vi "KPRO_2016_DPT.vi"() -> ()   [LabVIEW 2016]
uses:
  Kpro Globals.vi
  ad interface/Global_SIM_switch.vi
  <vilib>/Utility/file.llb/Write To Spreadsheet File (DBL).vi
panel:
  in  "Case Constant\n(See Context Help)":bool
  in  "Record DTW":bool
  out "Depth to Water":dbl=-30.877198474121087 format="%.2f"
  in  "In-Line Pressure Offset":dbl format="%.2f"
  in  "Zero In-Line Pressure\n(F = leave as is)":bool=TRUE
  in  "In-Line Pressure Slope":dbl=42.0 format="%.2f"
  out "In-Line Pressure":dbl=69.7228 format="%.2f"
  out "Drive Rate":dbl=16.666666666666664 format="%.2f"
  out "Real Time - Depth vs. Drive":cluster{dbl[], dbl[]}(graph)={[0.02036245163917736, 0.125, 0.16666666666666674, 0.16666666666666663, 0.16666666666666663, 0.16666666666666663], [-100.1, -100.2, -100.3, -100.4, -100.5, -100.6]}
  out "Current Depth (m)":sgl=-30.661383 format="%.2f"
  out "Zeroed \nPressure (m)":dbl=22.78027421497274 format="%.2f"
  out "Ik":dbl=0.003788962123473114 format="%.2f"
  in  "KPRO_test_report_header":string="Time(msecs)\tUncorrected_Depth\tCorrected_Depth\tDrive_Rate\tFlow\tFeet_of_Stainless\tPressure\tIK\tCorrected_Pressure\tAtm_Pressure\tDepth_to_water\tHeight_of_box\tRes_Pressure\tSecs_since_1_JAN_1904\tDepth_jumps_more_than_1_foot\r\n"
  in  "SLUG_test_report_header":string="Time(msecs)\tPressure\tFlow\n"
  in  "YSI_test_report_header":string="Depth\tPressure\tTemperature\tSpecific Conductivity\tDissolved O2\tPH\tOrp\tION\n"
  out "IK_for_GMS_report_header":string="Name\tHOLE_001\rXYZ\t20\t10\t30\rNumcols\t2\rNumrows\t1\rDepth\tIk\r"
  in  "Numrowswrite":string="1"
  in  "E":string="30"
  in  "Northing":string="10"
  in  "Easting":string="20"
  in  "Hole Id":string="HOLE_001"
  in  "Hole_name_file":path=path "C:/e"
  in  "Output File KPRO Test":path=path "C:/e_KPRO.txt"
  in  "Output File Slug Test":path=path "C:/e_SLUG.txt"
  in  "Output File YSI Test":path=path "C:/e_YSI.txt"
  in  "Output File IK for GMS":path=path "C:/e_IKMGS.txt"
  in  "enable_IKMGS_file":bool
  in  "enable_YSI_file":bool
  in  "enable_slug_file":bool
  in  "enable_kpro_file":bool=TRUE
  out "Ik":dbl=0.003788962123473114 format="%.2f"
  out "Zeroed Pressure":dbl=74.74207969932556 format="%.2f"
  out "Current Depth":sgl=-100.6 format="%.2f"
  out "Flow":dbl=0.21081600494384767 format="%.2f"
  out "Real Time - Depth vs. lk":cluster{dbl[], dbl[]}(graph)={[0.003788962123473114, 0.0037174584307500765, 0.0037174584307500765, 0.0037174584307500765, 0.0037174584307500765, 0.003788962123473114], [-100.1, -100.2, -100.3, -100.4, -100.5, -100.6]}
  out "Profile ID":string="WP-01"
  out "KPRO Box Number":dbl=800.0
  out "Last_String_Pot_Slope":dbl=1.6619999408721924 format="%.2f"
  out "Last_Flow_Slope":dbl=39.040000915527344 format="%.2f"
  out "Last_Pressure_Slope":dbl=48.27000045776367 format="%.2f"
  out "Height of Sample Box":dbl format="%.2f"
  out "Hole_Name_Path":path=path "C:/e"
  out "Cumulative_data_from_file":sgl[][](array[numeric]) format="%.2f"
  in  "data_directory":string="C:\\KPRO_DATA\\SITE_NAME\\"
  out "Cumulative_data_ready":bool
  out "Real Time - Depth vs. lk":cluster{dbl[], dbl[]}(graph)={[0.003788962123473114, 0.0037174584307500765, 0.0037174584307500765, 0.0037174584307500765, 0.0037174584307500765, 0.003788962123473114], [-100.1, -100.2, -100.3, -100.4, -100.5, -100.6]}
  in  "Reservoir Pressure":dbl=-0.004827000045779073 format="%.2f"
  in  "Simulate AD6B":bool
  in  "Atmospheric Pressure":dbl=32.22022530555725 format="%.2f"
  out "Depth to Water Table":dbl=-0.0 format="%.2f"
  in  "Ion Offset":dbl format="%.2f"
  in  "Ion Slope":dbl=44.04 format="%.2f"
  out "Pressure Slope":dbl=48.27000045776367 format="%.2f"
  out "Flow Slope":dbl=39.040000915527344 format="%.2f"
  out "String Pot Slope":dbl=1.6619999408721924 format="%.2f"
  in  "KPRO Com Port":i32=6
  in  "YSI Time Out (secs)":i32=5000
  in  "YSI Com Port":i32=7
  out "numrows":dbl format="%.2f"
  out "Slug Test\nIndicator copy":bool
  in  "ISE":bool=TRUE
  in  "Start\nYSI Capture":bool
  in  "Capture Head \nPressure":bool
  in  "Depth mode":bool caption="Use \nIncrement"
  out "Real Time - Depth vs. Drive":cluster{dbl[], dbl[]}(graph)={[0.02036245163917736, 0.125, 0.16666666666666674, 0.16666666666666663, 0.16666666666666663, 0.16666666666666663], [-100.1, -100.2, -100.3, -100.4, -100.5, -100.6]}
  out "Cumulative - Depth vs. Drive":cluster{dbl[], dbl[]}(graph)
  in  "Feet of Stainless":i32=40
  out "Zero Pressure\nIndicator":bool
  out "Slug Test\nIndicator":bool
  out "KPRO Test\nIndicator":bool
  in  "Increment\nButton":bool
  in  "Start\nST":bool
  in  "Zero\nPressure":bool
  out "Zeroed \nPressure":dbl=74.74207969932556 format="%.2f"
  in  "Finish Tests":bool
  out "Current Depth":sgl=-100.6 format="%.2f"
  in  "Start\nKPRO":bool
  out "Total Volume":dbl format="%.2f"
  in  "Clear \nTotal\nVolume":bool
  in  "Start Depth":sgl format="%.2f"
  in  "Client ID - Not Used":string
  out "Flow":dbl=0.21081600494384767 format="%.2f"
  out "Cumulative - Depth vs. Ik":cluster{dbl[], dbl[]}(graph)
  # "Use new slope/offset"
  # "KPRO  DATALOGGER"
  # "STONE  ENVIRONMENTAL  2010"
  # "ON"
  # "ON"
  # "OFF"
  # "OFF"
  # "ON"
  # "ON"
  # "OFF"
  # "OFF"
  # "ON"
  # "OFF"
  # "String Pot"
  # "Revision History\n\nAdded metric depth and pressure - VLD - 12-20-07\nAdded Static Ik button and drive rate- VLD 1-28-10"
  # "Use Incr"
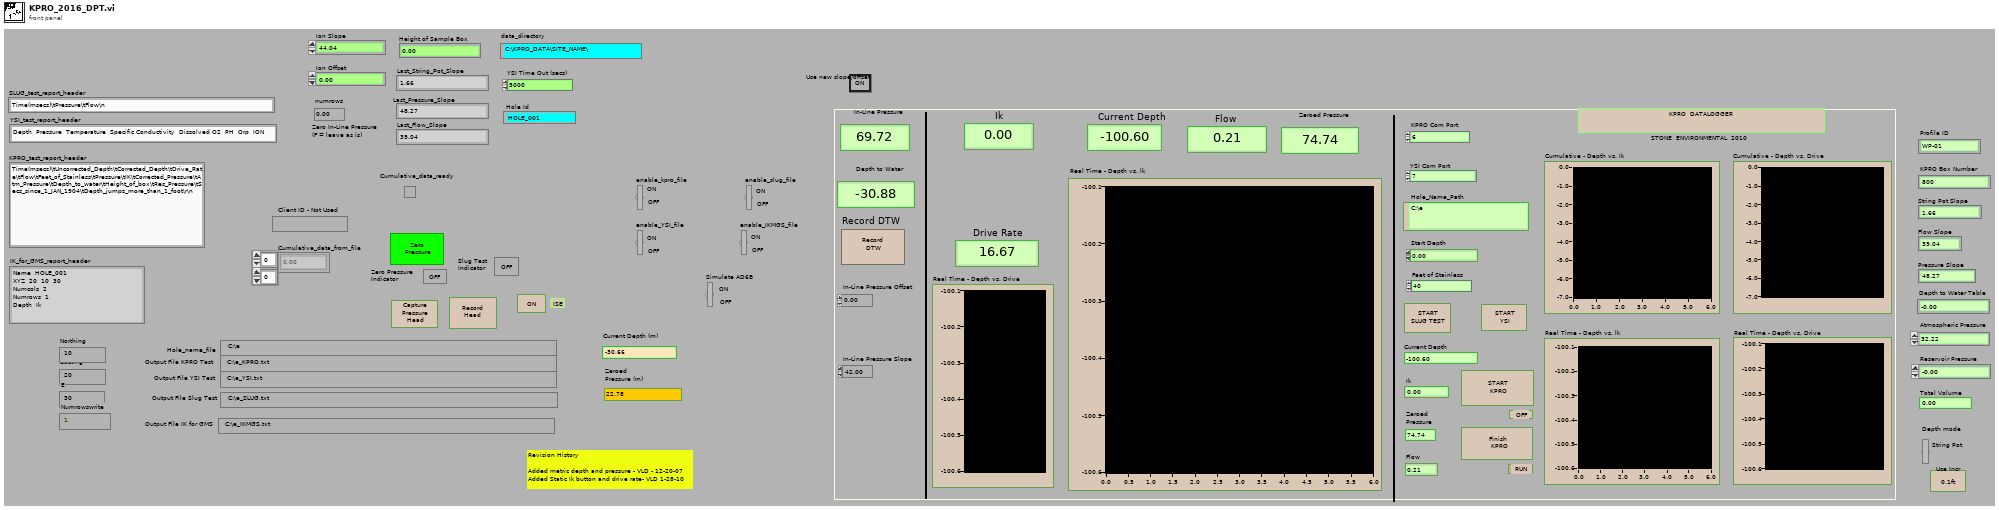
[diagram p1: front panel]
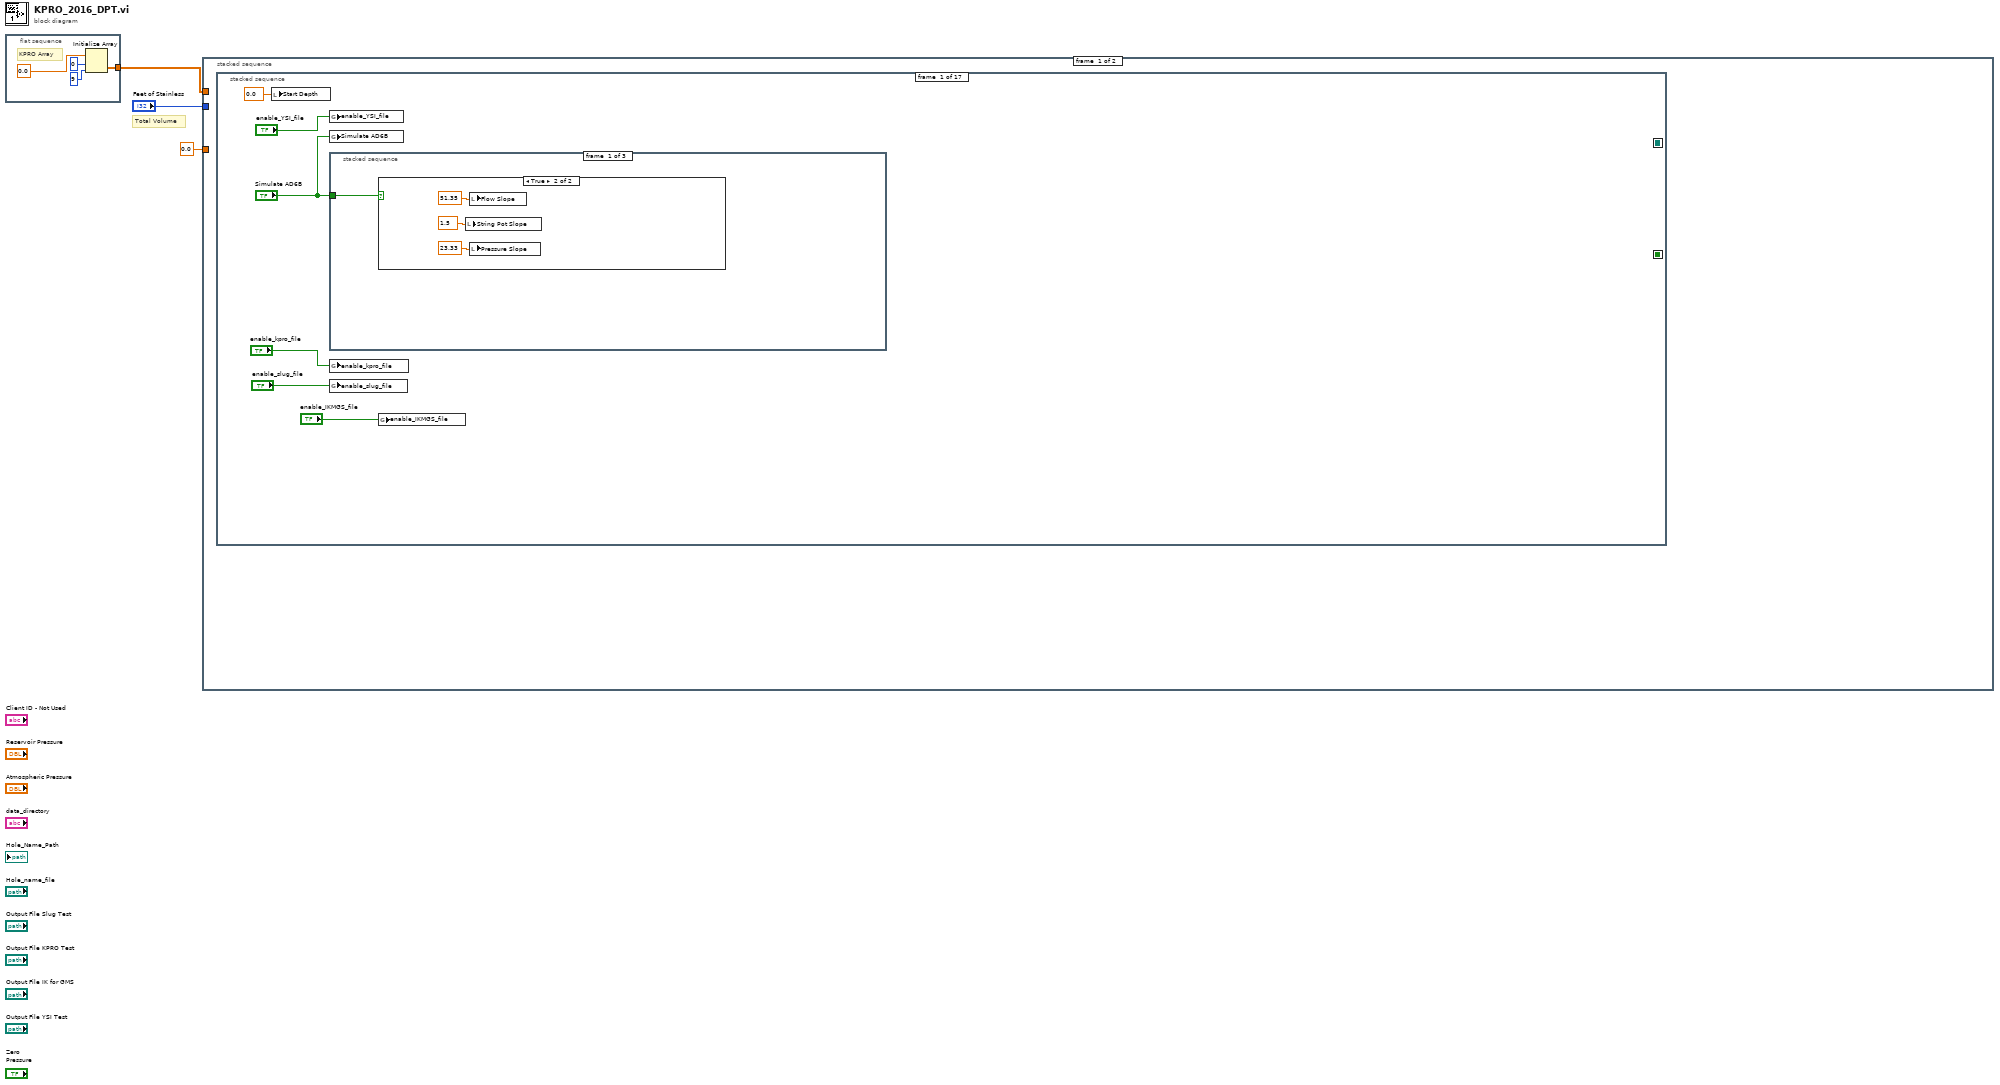
[diagram p0: block diagram]
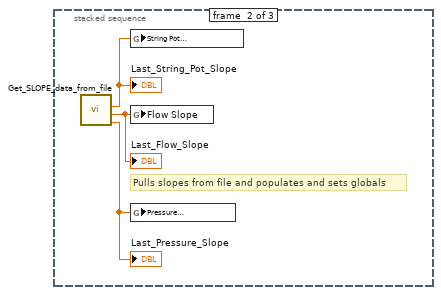
[diagram p3: hidden frame]
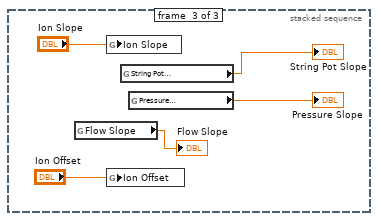
[diagram p4: hidden frame]
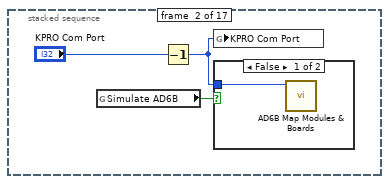
[diagram p5: hidden frame]
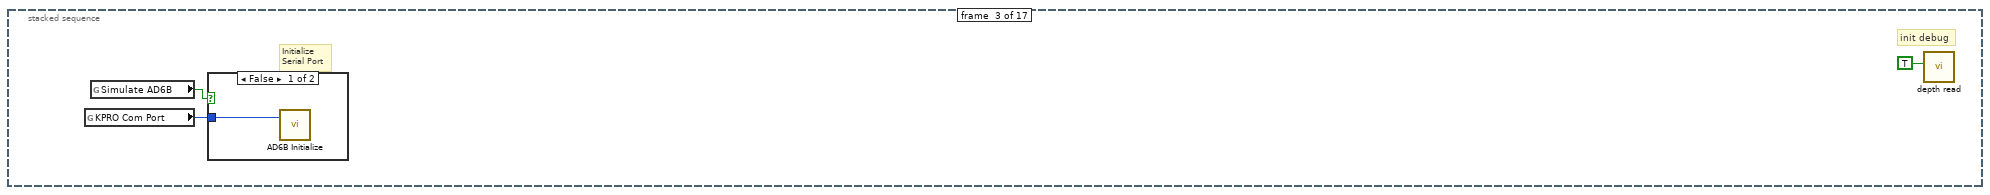
[diagram p7: hidden frame]
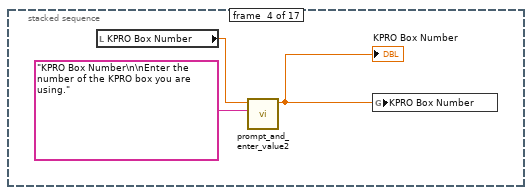
[diagram p9: hidden frame]
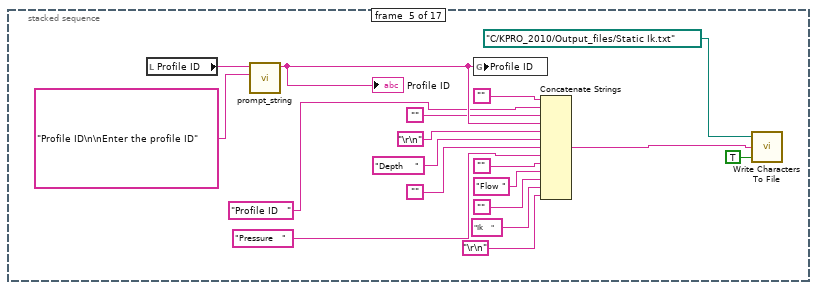
[diagram p10: hidden frame]
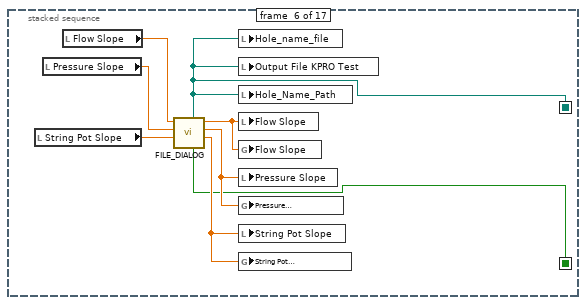
[diagram p11: hidden frame]
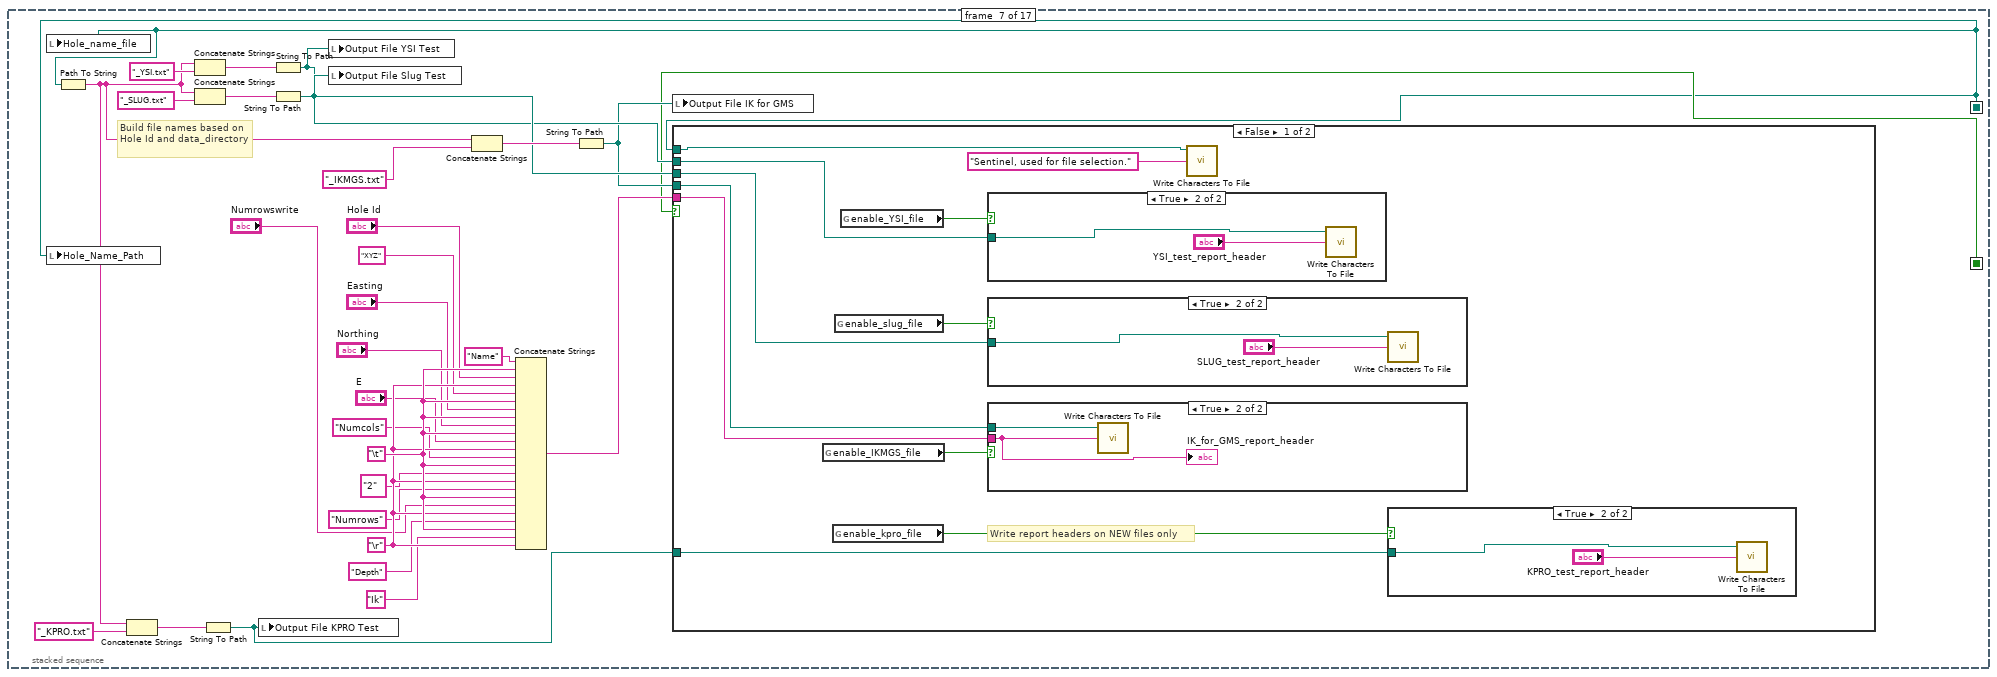
[diagram p12: hidden frame]
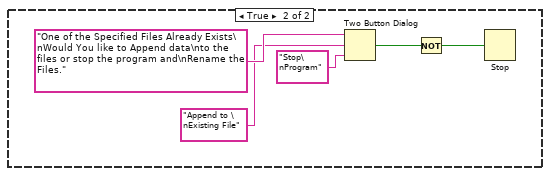
[diagram p17: hidden frame]
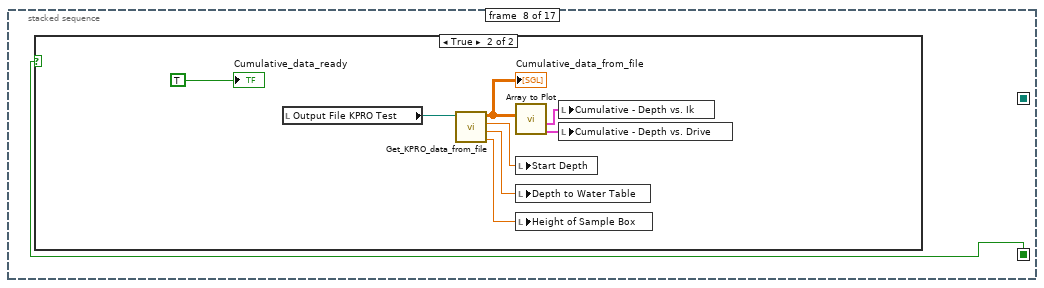
[diagram p18: hidden frame]
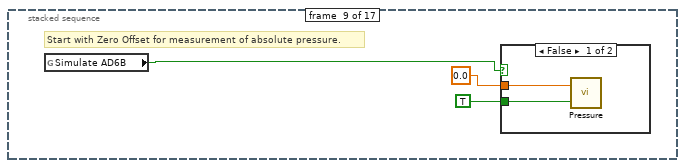
[diagram p20: hidden frame]
diagram:
  # "Total Volume"
  n1 = flat-sequence {
    tunnel: [w4] -> w1
    frame #0 {
      # "KPRO Array"
      n2 = Initialize Array(0.0, 0, 9) -> (w4:dbl[][])
    }
  }
  n3 = stacked-sequence {
    tunnel: "Feet of Stainless" -> [_ w195]
    tunnel: 0.0 -> [_ w194]
    tunnel: w1 -> [_ w193]
    frame #0 {
      n4 = stacked-sequence {
        seq-local: [_ _ _ _ _ w55 _ _ _ _ _ _ _ _ _ _ _] -> [_ _ _ _ _ _ w64 w117 _ _ _ _ _ _ _ _ _]
        seq-local: [_ _ _ _ _ w56 _ _ _ _ _ _ _ _ _ _ _] -> [_ _ _ _ _ _ w63 _ _ _ _ _ _ _ _ _ _]
        frame #0 {
          n5 = local write "Start Depth"(sgl 0.0 ("Start Depth")) -> ()
          n6 = global write "Global_SIM_switch.vi" "enable_YSI_file"("enable_YSI_file") -> ()
          n7 = global write "Global_SIM_switch.vi" "Simulate AD6B"("Simulate AD6B") -> ()
          n8 = stacked-sequence {
            tunnel: "Simulate AD6B" -> [w14 _ _]
            frame #0 {
              n9 = case shown="True" w14 {
                frame False {
                }
                frame True {
                  n10 = local write "String Pot Slope"(1.5 ("String Pot Slope")) -> ()
                  n11 = local write "Flow Slope"(51.35 ("Flow Slope")) -> ()
                  n12 = local write "Pressure Slope"(23.33 ("Pressure Slope")) -> ()
                }
              }
            }
            frame #1 {
              # "Pulls slopes from file and populates and sets globals"
              n13 = call "Get_SLOPE_data_from_file.vi"() -> ("Last_Pressure_Slope"=w20:dbl, "Last_Flow_Slope"=w19:dbl, "Last_String_Pot_Slope"=w18:dbl)  [unwired: 8 in, 1 out]
              "Last_Pressure_Slope" <- w20
              "Last_Flow_Slope" <- w19
              "Last_String_Pot_Slope" <- w18
              n14 = global write "Kpro Globals.vi" "String Pot \nSlope"(w18) -> ()
              n15 = global write "Kpro Globals.vi" "Flow Slope"(w19) -> ()
              n16 = global write "Kpro Globals.vi" "Pressure \nSlope"(w20) -> ()
            }
            frame #2 {
              n17 = global read "Kpro Globals.vi" "Flow Slope"() -> (→"Flow Slope":dbl)
              n18 = global write "Kpro Globals.vi" "Ion Slope"("Ion Slope") -> ()
              n19 = global write "Kpro Globals.vi" "Ion Offset"("Ion Offset") -> ()
              n20 = global read "Kpro Globals.vi" "String Pot \nSlope"() -> (→"String Pot Slope":dbl)
              n21 = global read "Kpro Globals.vi" "Pressure \nSlope"() -> (→"Pressure Slope":dbl)
            }
          }
          n22 = global write "Global_SIM_switch.vi" "enable_kpro_file"("enable_kpro_file") -> ()
          n23 = global write "Global_SIM_switch.vi" "enable_slug_file"("enable_slug_file") -> ()
          n24 = global write "Global_SIM_switch.vi" "enable_IKMGS_file"("enable_IKMGS_file") -> ()
        }
        frame #1 {
          n25 = global read "Global_SIM_switch.vi" "Simulate AD6B"() -> (w26:bool)
          n26 = Decrement(x="KPRO Com Port") -> (x-1=w27:i32)
          n27 = global write "Kpro Globals.vi" "KPRO Com Port"(w27) -> ()
          n28 = case shown="False" w26 {
            tunnel: w27 -> [w29 _]
            frame False {
              n29 = call "AD6B Map Modules & Boards.VI"("port number (1:com2)"=w29) -> ()  [unwired: 3 in, 3 out]
            }
            frame True {
            }
          }
        }
        frame #2 {
          # "init debug"
          # "Initialize\nSerial Port"
          n30 = global read "Kpro Globals.vi" "KPRO Com Port"() -> (w30:i32)
          n31 = global read "Global_SIM_switch.vi" "Simulate AD6B"() -> (w31:bool)
          n32 = case shown="False" w31 {
            tunnel: w30 -> [w33 _]
            frame False {
              n33 = call "AD6B Initialize.VI"("port number (1:com2)"=w33) -> ()  [unwired: 2 in, 1 out]
            }
            frame True {
            }
          }
          n34 = call "depth read.vi"("Initialize Debug"=TRUE) -> ()  [unwired: 3 in, 1 out]
        }
        frame #3 {
          n35 = local read "KPRO Box Number"() -> (w34:dbl)
          n36 = call "prompt_and_enter_value2.vi"("prompt_IN"="KPRO Box Number\n\nEnter the number of the KPRO box you are using." ("prompt"), "Enter value"=w34) -> ("Numeric"=w35:dbl)  [unwired: 9 in]
          "KPRO Box Number" <- w35
          n37 = global write "Kpro Globals.vi" "KPRO Box Number"(w35) -> ()
        }
        frame #4 {
          n38 = local read "Profile ID"() -> (w54:string)
          n39 = call "prompt_string.vi"("prompt_IN"="Profile ID\n\nEnter the profile ID" ("prompt"), "Enter value"=w54) -> ("String"=w50:string)  [unwired: 9 in]
          "Profile ID" <- w50
          n40 = global write "Kpro Globals.vi" "Profile ID"(w50) -> ()
          n41 = Concatenate Strings("" ("string"), "Profile ID   " ("string"), "" ("string"), w50, "\r\n", "Depth    " ("string"), "" ("string"), "Pressure   " ("string"), "" ("string"), "Flow " ("string"), "" ("string"), "Ik    " ("string"), "\r\n") -> (w49:string)
          n42 = call <vilib>:"Write Characters To File.vi"("append to file? (new file:F)"=TRUE, "character string"=w49, "file path (dialog if empty)"=path "C:/KPRO_2010/Output_files/Static Ik.txt") -> ()  [unwired: 2 in, 1 out]
        }
        frame #5 {
          n43 = local read "String Pot Slope"() -> (w60:dbl)
          n44 = local read "Pressure Slope"() -> (w61:dbl)
          n45 = local read "Flow Slope"() -> (w62:dbl)
          n46 = call "FILE_DIALOG.vi"("string_pot_slope_IN"=w60, "pressure_slope_IN"=w61, "flow_slope_IN"=w62) -> ("string_pot_slope_OUT"=w57:dbl, "pressure_slope_OUT"=w58:dbl, "flow_slope_OUT"=w59:dbl, "exists"=w55:bool, "path"=w56:path)  [unwired: 3 in, 1 out]
          n47 = local write "Hole_name_file"(w56) -> ()
          n48 = local write "Output File KPRO Test"(w56) -> ()
          n49 = local write "Hole_Name_Path"(w56) -> ()
          n50 = local write "Flow Slope"(w59) -> ()
          n51 = global write "Kpro Globals.vi" "Flow Slope"(w59) -> ()
          n52 = local write "Pressure Slope"(w58) -> ()
          n53 = global write "Kpro Globals.vi" "Pressure \nSlope"(w58) -> ()
          n54 = local write "String Pot Slope"(w57) -> ()
          n55 = global write "Kpro Globals.vi" "String Pot \nSlope"(w57) -> ()
        }
        frame #6 {
          w92 = "\t"
          w91 = "\r" ("Carriage Return")
          # "Build file names based on Hole Id and data_directory"
          n56 = local write "Hole_name_file"(w63) -> ()
          n57 = local write "Hole_Name_Path"(w63) -> ()
          n58 = Path To String(path=w63) -> (string=w74:string)
          n59 = Concatenate Strings(w74, "_KPRO.txt") -> (w80:string)
          n60 = Concatenate Strings(w74, "_YSI.txt") -> (w78:string)
          n61 = Concatenate Strings(w74, "_SLUG.txt") -> (w79:string)
          n62 = String To Path(string=w80) -> (path=w73:path)
          n63 = local write "Output File KPRO Test"(w73) -> ()
          n64 = String To Path(string=w78) -> (path=w71:path)
          n65 = String To Path(string=w79) -> (path=w72:path)
          n66 = local write "Output File YSI Test"(w71) -> ()
          n67 = local write "Output File Slug Test"(w72) -> ()
          n68 = Concatenate Strings(w74, "_IKMGS.txt") -> (w77:string)
          n69 = Concatenate Strings("Name" ("Name"), w92, "Hole Id", w91, "XYZ" ("date string"), w92, "Easting", w92, "Northing", w92, "E", w91, "Numcols", w92, "2", w91, "Numrows", w92, "Numrowswrite", w91, "Depth", w92, "Ik", w91) -> (w83:string)
          n70 = String To Path(string=w77) -> (path=w70:path)
          n71 = local write "Output File IK for GMS"(w70) -> ()
          n72 = case shown="False" w64 {
            tunnel: w83 -> [w97 _]
            tunnel: w63 -> [w102 _]
            tunnel: w73 -> [w101 _]
            tunnel: w72 -> [w100 _]
            tunnel: w71 -> [w99 _]
            tunnel: w70 -> [w98 _]
            frame False {
              # "Write report headers on NEW files only"
              n73 = global read "Global_SIM_switch.vi" "enable_IKMGS_file"() -> (w93:bool)
              n74 = global read "Global_SIM_switch.vi" "enable_kpro_file"() -> (w96:bool)
              n75 = global read "Global_SIM_switch.vi" "enable_slug_file"() -> (w95:bool)
              n76 = global read "Global_SIM_switch.vi" "enable_YSI_file"() -> (w94:bool)
              n77 = case shown="True" w94 {
                tunnel: w99 -> [_ w107]
                frame False {
                }
                frame True {
                  n78 = call <vilib>:"Write Characters To File.vi"("character string"="YSI_test_report_header", "file path (dialog if empty)"=w107) -> ()  [unwired: 3 in, 1 out]
                }
              }
              n79 = case shown="True" w95 {
                tunnel: w100 -> [_ w109]
                frame False {
                }
                frame True {
                  n80 = call <vilib>:"Write Characters To File.vi"("character string"="SLUG_test_report_header", "file path (dialog if empty)"=w109) -> ()  [unwired: 3 in, 1 out]
                }
              }
              n81 = case shown="True" w93 {
                tunnel: w98 -> [_ w105]
                tunnel: w97 -> [_ w104]
                frame False {
                }
                frame True {
                  n82 = call <vilib>:"Write Characters To File.vi"("character string"=w104, "file path (dialog if empty)"=w105) -> ()  [unwired: 3 in, 1 out]
                  "IK_for_GMS_report_header" <- w104
                }
              }
              n83 = call <vilib>:"Write Characters To File.vi"("character string"="Sentinel, used for file selection.", "file path (dialog if empty)"=w102) -> ()  [unwired: 3 in, 1 out]
              n84 = case shown="True" w96 {
                tunnel: w101 -> [_ w111]
                frame False {
                }
                frame True {
                  n85 = call <vilib>:"Write Characters To File.vi"("character string"="KPRO_test_report_header", "file path (dialog if empty)"=w111) -> ()  [unwired: 3 in, 1 out]
                }
              }
            }
            frame True {
              n86 = Two Button Dialog(message="One of the Specified Files Already Exists\nWould You like to Append data\nto the files or stop the program and\nRename the Files.", 1:"Stop\nProgram", 2:"Append to \nExisting File") -> (T button?=w112:bool)
              n87 = Not(x=w112) -> (.not. x?=w113:bool)
              n88 = Stop(stop? (T)=w113) -> ()
            }
          }
        }
        frame #7 {
          n89 = case shown="True" w117 {
            frame False {
            }
            frame True {
              n90 = local read "Output File KPRO Test"() -> (w121:path)
              n91 = call "Get_KPRO_data_from_file.vi"("Output File KPRO Test"=w121) -> ("Last_height_of_box"=w118:dbl, "Last_depth_to_water"=w119:dbl, "Last_depth"=w125:dbl, "Output_array"=w122:sgl[][])  [unwired: 7 in]
              "Cumulative_data_from_file" <- w122
              n92 = call "Array to Plot.vi"("Input Cumulative Array"=w122) -> ("Cumulative - Depth vs.Drive Rate"=w123:cluster{dbl[], dbl[]}, "Cumulative - Depth vs. Ik"=w124:cluster{dbl[], dbl[]})  [unwired: 3 in, 4 out]
              n93 = local write "Start Depth"(w125) -> ()
              n94 = local write "Depth to Water Table"(w119) -> ()
              n95 = local write "Height of Sample Box"(w118) -> ()
              n96 = local write "Cumulative - Depth vs. Ik"(w124) -> ()
              n97 = local write "Cumulative - Depth vs. Drive"(w123) -> ()
              "Cumulative_data_ready" <- TRUE ("Cumulative_data_ready")
            }
          }
        }
        frame #8 {
          # "Start with Zero Offset for measurement of absolute pressure."
          n98 = global read "Global_SIM_switch.vi" "Simulate AD6B"() -> (w126:bool)
          n99 = case shown="False" w126 {
            tunnel: TRUE -> [w129 w131]
            tunnel: 0.0 -> [w130 w132]
            frame False {
              n100 = call "Pressure.vi"("Zero Pressure\n(F = leave as is)"=w129, "Pressure Offset"=w130) -> ()  [unwired: 1 in, 1 out]
            }
            frame True {
              n101 = call "SIM_Pressure.vi"("Zero Pressure\n(F = leave as is)"=w131, "Pressure Offset"=w132) -> ()  [unwired: 9 in, 1 out]
            }
          }
        }
        frame #9 {
          # "Take offset and put\n into Pressure VI."
          n102 = global read "Global_SIM_switch.vi" "Simulate AD6B"() -> (w134:bool)
          n103 = call "PRESSURE_CAL.vi"("sim_low"=29.9 ("sim_high"), "sim_high"=29.96, "Prompt_IN"="ATMOSPHERIC PRESSURE READING\n\nHold Kpro effluent facing up and level with the pressure transducer.\nTurn on Kpro water, turn off when water flows with no air bubbles.\n\nPress OK when the reading equilibrates." ("message")) -> ("PRESSURE\nFt of water"=w133:dbl)  [unwired: 8 in]
          n104 = global write "Kpro Globals.vi" "Atmospheric Pressure"(w133) -> ()
          n105 = local write "Atmospheric Pressure"(w133) -> ()
          n106 = case shown="False" w134 {
            tunnel: w133 -> [w140 w142]
            tunnel: TRUE -> [w139 w141]
            frame False {
              n107 = call "Pressure.vi"("Zero Pressure\n(F = leave as is)"=w139, "Pressure Offset"=w140) -> ()  [unwired: 1 in, 1 out]
            }
            frame True {
              n108 = call "SIM_Pressure.vi"("Zero Pressure\n(F = leave as is)"=w141, "Pressure Offset"=w142) -> ()  [unwired: 9 in, 1 out]
            }
          }
        }
        frame #10 {
          n109 = case shown="True" "Case Constant\n(See Context Help)" {
            frame False {
            }
            frame True {
              # "Take offset and put\n into Pressure VI."
              n110 = call "PRESSURE_CAL.vi"("sim_low"=30.9 ("sim_high"), "sim_high"=30.96, "Prompt_IN"="ZERO PRESSURE TRANSDUCER\n\nHold Kpro effluent in a grad cylinder with 800mL (1 ft) of water.\nHold grad cylinder with its bottom level with the pressure transducer.\n\nPress OK when the reading equilibrates. " ("message")) -> ("PRESSURE\nFt of water"=w144:dbl)  [unwired: 8 in]
              n111 = global read "Global_SIM_switch.vi" "Simulate AD6B"() -> (w146:bool)
              n112 = Subtract(x=w144, y=1.0) -> (x-y=w148:dbl)
              n113 = case shown="False" w146 {
                tunnel: [w153 w154] -> w147
                frame False {
                  n114 = call "Flow.vi"() -> ("Flow (ml/min)"=w153:dbl)  [unwired: 3 in]
                }
                frame True {
                  n115 = call "SIM_Flow.vi"() -> ("Flow (ml/min)"=w154:dbl)  [unwired: 3 in]
                }
              }
              n116 = case shown="False" w146 {
                tunnel: w148 -> [w156 w158]
                tunnel: TRUE -> [w155 w157]
                frame False {
                  n117 = call "Pressure.vi"("Zero Pressure\n(F = leave as is)"=w155, "Pressure Offset"=w156) -> ()  [unwired: 1 in, 1 out]
                }
                frame True {
                  n118 = call "SIM_Pressure.vi"("Zero Pressure\n(F = leave as is)"=w157, "Pressure Offset"=w158) -> ()  [unwired: 9 in, 1 out]
                }
              }
              n119 = local write "Flow"(w147) -> ()
            }
          }
        }
        frame #11 {
          n120 = call "PRESSURE_CAL.vi"("sim_low"=99.5 ("sim_high"), "sim_high"=100.5, "Prompt_IN"="CHECK RESERVOIR PRESSURE\n\nTurn on Kpro. Unplug Kpro Out quick connect from sample box.\nReservoir pressure should be 69.2 +/- 5%(65.7 - 72.7).\n\nPress OK when the reading equilibrates within range." ("message")) -> ("PRESSURE\nFt of water"=w161:dbl)  [unwired: 8 in]
          n121 = local write "Reservoir Pressure"(w161) -> ()
          n122 = global write "Kpro Globals.vi" "Reservoir Pressure"(w161) -> ()
        }
        frame #12 {
          n123 = local read "Start Depth"() -> (w167:sgl)
          n124 = call "prompt_and_enter_value.vi"("prompt_IN"="ENTER START DEPTH", "Enter value"=w167) -> ("Numeric"=w165:dbl)  [unwired: 9 in]
          n125 = Absolute Value(x=w165) -> (abs(x)=w164:dbl)
          n126 = Negate(x=w164) -> (-x=w163:dbl)
          n127 = local write "Start Depth"(w163) -> ()
        }
        frame #13 {
          n128 = local read "Height of Sample Box"() -> (w169:dbl)
          n129 = call "prompt_and_enter_value.vi"("prompt_IN"="HEIGHT FROM GROUND SURFACE TO SAMPLE BOX\n\nMeasure the vertical distance between the ground surface and the pressure transducer." ("prompt"), "Enter value"=w169) -> ("Numeric"=w168:dbl)  [unwired: 9 in]
          "Height of Sample Box" <- w168
          n130 = global write "Kpro Globals.vi" "height_of_box"(w168) -> ()
        }
        frame #14 {
          n131 = local read "Depth to Water Table"() -> (w174:dbl)
          n132 = call "prompt_and_enter_value.vi"("prompt_IN"="DEPTH TO WATER TABLE\n\nEnter the depth to the water table." ("prompt"), "Enter value"=w174) -> ("Numeric"=w173:dbl)  [unwired: 9 in]
          n133 = Absolute Value(x=w173) -> (abs(x)=w172:dbl)
          n134 = Negate(x=w172) -> (-x=w171:dbl)
          "Depth to Water Table" <- w171
          n135 = global write "Kpro Globals.vi" "Depth to Water Table"(w171) -> ()
        }
        frame #15 {
          n136 = stacked-sequence {
            frame #0 {
              # "Set to raw pressure mode"
              n137 = global read "Global_SIM_switch.vi" "Simulate AD6B"() -> (w177:bool)
              n138 = case shown="False" w177 {
                tunnel: TRUE -> [w178 w180]
                frame False {
                  n139 = call "Pressure.vi"("Zero Pressure\n(F = leave as is)"=w178, "Pressure Offset"=0.0) -> ()  [unwired: 1 in, 1 out]
                }
                frame True {
                  n140 = call "SIM_Pressure.vi"("Zero Pressure\n(F = leave as is)"=w180) -> ()  [unwired: 10 in, 1 out]
                }
              }
            }
            frame #1 {
              # "adjust for 1 foot head"
              # "Take offset and put\n into Pressure VI."
              n141 = call "PRESSURE_CAL.vi"("sim_low"=29.9 ("sim_high"), "sim_high"=29.96, "Prompt_IN"="ZERO TO GROUND SURFACE\n\nFill a grad cylinder to 750mL.\nPlace it on the ground at the profile location.\nImmerse the Kpro effluent and turn on Kpro flow.\nTurn off after water is flowing with no bubbles\nand the water has reached 800mL (1 foot).\n\nPress OK when the reading equilibrates." ("message")) -> ("PRESSURE\nFt of water"=w181:dbl)  [unwired: 8 in]
              n142 = Decrement(x=w181) -> (x-1=w182:dbl)
              n143 = global read "Global_SIM_switch.vi" "Simulate AD6B"() -> (w184:bool)
              n144 = case shown="False" w184 {
                tunnel: w182 -> [w189 w191]
                tunnel: TRUE -> [w188 w190]
                frame False {
                  n145 = call "Pressure.vi"("Zero Pressure\n(F = leave as is)"=w188, "Pressure Offset"=w189) -> ()  [unwired: 1 in, 1 out]
                }
                frame True {
                  n146 = call "SIM_Pressure.vi"("Zero Pressure\n(F = leave as is)"=w190, "Pressure Offset"=w191) -> ()  [unwired: 9 in, 1 out]
                }
              }
            }
          }
        }
        frame #16 {
          n147 = flat-sequence {
            frame #0 {
              w192 = FALSE
              n148 = local write "Slug Test\nIndicator"(w192) -> ()
              n149 = local write "KPRO Test\nIndicator"(w192) -> ()
              "Zero Pressure\nIndicator" <- w192
            }
          }
        }
      }
    }
    frame #1 {
      # "End"
      # "State"
      n150 = while {
        shift-left: w193 -> [w204]
        shift-right: [w203] -> _
        shift-left: w195 -> [w206]
        shift-right: [w205] -> _
        shift-left: _ -> [w209]
        shift-right: [w208] -> _
        shift-left: w194 -> [w207]
        shift-right: [w202] -> _
        shift-left: TRUE -> [w212]
        shift-right: [w211] -> _
        shift-left: 0 -> [w213]
        shift-right: [w210] -> _
        stop <- TRUE continue-if-true
        n151 = Wait (ms)(milliseconds to wait=u32 200) -> ()  [unwired: 1 out]
        n152 = call "bool debounce.vi"("Input Boolean"="Finish Tests") -> ("Output Boolean"=w200:bool)
        "Slug Test\nIndicator copy" <- w200
        n153 = stacked-sequence {
          seq-local: [_ w243 _] -> [_ _ w275]
          seq-local: [_ w254 _] -> [_ _ w274]
          seq-local: [w221 _ _] -> [_ _ w272]
          seq-local: [w222 _ _] -> [_ _ w271]
          tunnel: w213 -> [_ w256 _]
          tunnel: w212 -> [_ w255 _]
          tunnel: [_ _ w276] -> w211
          tunnel: [_ w243 _] -> w210
          tunnel: w200 -> [_ _ w273]
          tunnel: w209 -> [_ _ w270]
          tunnel: [_ _ w269] -> w208
          tunnel: w207 -> [_ _ w268]
          tunnel: [_ _ w267] -> w202
          tunnel: w206 -> [_ _ w266]
          tunnel: [_ _ w265] -> w205
          tunnel: w204 -> [_ _ w264]
          tunnel: [_ _ w263] -> w203
          frame #0 {
            n154 = global read "Kpro Globals.vi" "Current Depth"() -> (w217:sgl)
            n155 = call "In-Line-Pressure.vi"("Zero Pressure\n(F = leave as is)"="Zero In-Line Pressure\n(F = leave as is)", "In-Line Pressure Slope"="In-Line Pressure Slope", "In-Line Pressure Offset"="In-Line Pressure Offset") -> ("Pressure"=w218:dbl)  [unwired: 1 in]
            "In-Line Pressure" <- w218
            n156 = Add(x=w218, y=w217) -> (x+y=w214:dbl)
            "Depth to Water" <- w214
            n157 = case shown="True" "Record DTW" {
              selector: "Record DTW" -> [w228 _]
              tunnel: [w228 FALSE ("Boolean")] -> _
              tunnel: w214 -> [_ w232]
              tunnel: w217 -> [_ w233]
              tunnel: "In-Line Pressure Offset" -> [_ w230]
              tunnel: w218 -> [_ w231]
              tunnel: "In-Line Pressure Slope" -> [_ w229]
              frame False {
              }
              frame True {
                n158 = Build Array(w233, w232, w231, w230, w229) -> (w237:dbl[])
                n159 = call-poly <vilib>:"Write To Spreadsheet File.vi"("append to file? (new file:F)"=TRUE, "1D data"=w237, "file path (dialog if empty)"=path "C:/KPRO_2010/Output_files/DTW.txt") -> ()  [unwired: 5 in, 1 out]
              }
            }
            n160 = global read "Global_SIM_switch.vi" "Simulate AD6B"() -> (w223:bool)
            n161 = case shown="False" w223 {
              tunnel: [w240 w242] -> w222
              tunnel: [w239 w241] -> w221
              frame False {
                n162 = call "Flow.vi"() -> ("Flow (ml/min)"=w240:dbl)  [unwired: 3 in]
                n163 = call "Pressure.vi"("Zero Pressure\n(F = leave as is)"=FALSE ("Zero Pressure\n(F = leave as is)")) -> ("Pressure"=w239:dbl)  [unwired: 2 in]
              }
              frame True {
                n164 = call "SIM_Flow.vi"() -> ("Flow (ml/min)"=w242:dbl)  [unwired: 3 in]
                n165 = call "SIM_Pressure.vi"() -> ("Pressure"=w241:dbl)  [unwired: 11 in]
              }
            }
            n166 = flat-sequence {
              tunnel: w222 -> [w224]
              frame #0 {
                "Flow" <- w224
                "Flow" <- w224
              }
            }
            n167 = flat-sequence {
              tunnel: w221 -> [w227]
              frame #0 {
                n168 = Divide(x=w227, y=3.281) -> (x/y=→"Zeroed \nPressure (m)":dbl)
                "Zeroed \nPressure" <- w227
                "Zeroed Pressure" <- w227
              }
            }
          }
          frame #1 {
            n169 = call "State Controller.vi"("Start KPRO"="Start\nKPRO", "Start Slug Test"="Start\nST", "Start YSI Capture"="Start\nYSI Capture", "Clear Volume"="Clear \nTotal\nVolume", "Capture Head Pressure"="Capture Head \nPressure", "Done"=w255, "Previous \nState"=w256) -> ("Next State"=w243:i32, "State Changed"=w254:bool, "Start KPRO Enabler"=w248:u8, "Start Slug Test Enabler"=w247:u8, "Start YSI Capture Enabler"=w246:u8, "Clear Volume Enabler"=w245:u8, "Capture Head Pressure Enabler"=w244:u8)  [unwired: 4 in, 2 out]
            n170 = property on="Start\nKPRO" class="Bool"("Disabled"=w248) -> ()  [unwired: 2 in, 2 out]
            n171 = property on="Start\nST" class="Bool"("Disabled"=w247) -> ()  [unwired: 2 in, 2 out]
            n172 = property on="Clear \nTotal\nVolume" class="Bool"("Disabled"=w245) -> ()  [unwired: 2 in, 2 out]
            n173 = flat-sequence {
              tunnel: w243 -> [w257]
              frame #0 {
                n174 = Equal?(x=w257, y=2) -> (x = y?=→"Slug Test\nIndicator":bool)
              }
            }
            n175 = flat-sequence {
              tunnel: w243 -> [w260]
              frame #0 {
                n176 = Equal?(x=w260, y=1) -> (x = y?=→"KPRO Test\nIndicator":bool)
              }
            }
            n177 = property on="Start\nYSI Capture" class="Bool"("Disabled"=w246) -> ()  [unwired: 2 in, 2 out]
            n178 = property on="Capture Head \nPressure" class="Bool"("Disabled"=w244) -> ()  [unwired: 2 in, 2 out]
          }
          frame #2 {
            # "Flow"
            # "Pressure"
            n179 = case shown="1" w275 {
              tunnel: [FALSE w304 w331 w338 TRUE TRUE] -> w276
              tunnel: w274 -> [_ w313 w331 w340 _ _]
              tunnel: w273 -> [_ w312 _ w339 _ _]
              tunnel: w272 -> [_ w311 _ _ _ w359]
              tunnel: w271 -> [_ w310 _ _ _ _]
              tunnel: w270 -> [_ w309 w332 w341 w356 w358]
              tunnel: [w277 w294 w332 w341 w356 w358] -> w269
              tunnel: w268 -> [w282 w308 w335 w344 _ w363]
              tunnel: [w282 w299 w335 w344 0.0 w363] -> w267
              tunnel: w266 -> [w281 w291 w333 w343 w354 w362]
              tunnel: [w281 w305 w333 w343 w354 w362] -> w265
              tunnel: w264 -> [w280 w298 w334 w342 w353 w361]
              tunnel: [w279 w302 w334 w342 w353 w361] -> w263
              frame 0, Default {
                # "Idle State"
                n180 = local read "Cumulative_data_ready"() -> (w278:bool)
                n181 = case shown="True" w278 {
                  tunnel: w280 -> [w288 _]
                  tunnel: [w288 w289] -> w279
                  frame False {
                  }
                  frame True {
                    n182 = local write "Cumulative_data_ready"(FALSE ("Get_KPRO_data")) -> ()
                    n183 = local read "Cumulative_data_from_file"() -> (w289:sgl[][])
                  }
                }
                n184 = flat-sequence {
                  tunnel: [w284] -> w277
                  frame #0 {
                    n185 = Less Or Equal To 0?(x="Start Depth") -> (x <= 0?=w287:bool)
                    n186 = Negate(x="Start Depth") -> (-x=w285:sgl)
                    n187 = Select(t="Start Depth", s=w287, f=w285) -> (s? t:f=w284:sgl)
                  }
                }
              }
              frame 1 {
                # "KPRO"
                n188 = flat-sequence {
                  frame #0 {
                    n189 = local read "numrows"() -> (→"numrows":dbl)
                  }
                }
                n190 = flat-sequence {
                  frame #0 {
                    n191 = global read "Kpro Globals.vi" "Depth to Water Table"() -> (w315:dbl)
                    n192 = local write "Depth to Water Table"(w315) -> ()
                  }
                }
                n193 = local read "Output File KPRO Test"() -> (w297:path)
                n194 = call "kpro.vi"("Output KPRO"=w297, "Initialize"=w313, "Finished In"=w312, "Absolute Depth In"=w309, "Total Volume in"=w308, "Zeroed Pressure"=w311, "Flow"=w310, "Read String Pot"="Depth mode", "Increment"="Increment\nButton", "SS In"=w291) -> ("Finished Out"=w304:bool, "SS Out"=w305:i32, "Current Depth Out"=w294:sgl, "Total Volume Out"=w299:dbl, "Output Array"=w303:dbl[][])  [unwired: 1 in]
                n195 = local write "Feet of Stainless"(w305) -> ()
                n196 = flat-sequence {
                  tunnel: w294 -> [w318]
                  frame #0 {
                    n197 = global write "Kpro Globals.vi" "Current Depth"(w318) -> ()
                    n198 = Divide(x=w318, y=3.281) -> (x/y=→"Current Depth (m)":dbl)
                    "Current Depth" <- w318
                    "Current Depth" <- w318
                  }
                }
                n199 = case shown="True" w304 {
                  tunnel: [w323 w330] -> w302
                  tunnel: w303 -> [_ w329]
                  tunnel: w298 -> [w323 w325]
                  frame False {
                  }
                  frame True {
                    n200 = Build Array (concatenate)(w325, w329) -> (w330:dbl[][])
                    n201 = global read "Kpro Globals.vi" "Current Depth"() -> (w324:sgl)
                    n202 = local read "Output File IK for GMS"() -> (w327:path)
                    n203 = local write "Start Depth"(w324) -> ()
                    n204 = call "IKGMS.vi"("format (%.3f)"="%.2F", "append to file? (new file:F)"=TRUE, "2D data"=w329, "file path (dialog if empty)"=w327) -> ()  [unwired: 4 in, 1 out]
                  }
                }
                n205 = call "Array to Plot.vi"("Input Cumulative Array"=w302, "Input Real Time Array"=w303) -> ("Cumulative - Depth vs.Drive Rate"=→"Cumulative - Depth vs. Drive":cluster{dbl[], dbl[]}, "Cumulative - Depth vs. Ik"=→"Cumulative - Depth vs. Ik":cluster{dbl[], dbl[]}, "Real Time - Depth vs. Drive Rate"=→"Real Time - Depth vs. Drive" →"Real Time - Depth vs. Drive":cluster{dbl[], dbl[]}, "Real Time - Depth vs. Ik"=→"Real Time - Depth vs. lk" →"Real Time - Depth vs. lk":cluster{dbl[], dbl[]}, "Current Ik"=w293:dbl, "Depth Rate"=w292:dbl)  [unwired: 2 in]
                n206 = flat-sequence {
                  tunnel: w292 -> [w321]
                  frame #0 {
                    n207 = Multiply(x=w321, y=100) -> (x*y=→"Drive Rate":dbl)
                  }
                }
                n208 = flat-sequence {
                  tunnel: w293 -> [w314]
                  frame #0 {
                    "Ik" <- w314
                    "Ik" <- w314
                  }
                }
              }
              frame 2 {
                n209 = flat-sequence {
                  tunnel: w333 -> [w337]
                  frame #0 {
                    n210 = local read "Output File Slug Test"() -> (w336:path)
                    n211 = call "Slug Test.vi"("# SS"=w337, "Output File"=w336) -> ()  [unwired: 10 in]
                  }
                }
              }
              frame 3 {
                n212 = flat-sequence {
                  tunnel: w341 -> [w351]
                  tunnel: w340 -> [w350]
                  tunnel: w339 -> [w349]
                  tunnel: [w348] -> w338
                  frame #0 {
                    n213 = call "Capture YSI.vi"("Initialize"=w350, "Finished In"=w349, "DEPTH"=w351, "YSI Com Port"="YSI Com Port", "Time Out (secs)"="YSI Time Out (secs)", "Collect Ion Data"="ISE") -> ("Finished Out"=w348:bool)  [unwired: 9 in]
                  }
                }
              }
              frame 4 {
              }
              frame 5 {
                n214 = global read "Global_SIM_switch.vi" "enable_YSI_file"() -> (w357:bool)
                n215 = case shown="True" w357 {
                  tunnel: w359 -> [_ w366]
                  tunnel: w358 -> [_ w365]
                  frame False {
                  }
                  frame True {
                    # "Capture Head Pressure"
                    n216 = local read "Output File YSI Test"() -> (w364:path)
                    n217 = call "Write YSI Data X.vi"("Output File"=w364, "Absolute Depth In"=w365, "Zeroed Pressure"=w366, "Update Pressure = False\nUpdate YSI = True"=FALSE) -> ()  [unwired: 12 in]
                  }
                }
              }
            }
          }
        }
      }
    }
  }
